vi "Error - Log.vi"(8 "error in (no error)":errorcluster, 11 "Error Data":T1) -> (0 "error out":errorcluster)   [LabVIEW 2017]
doc: "Maintainance a error log file\n[Covers: EH4]"
uses:
  Controls/Error Data.ctl
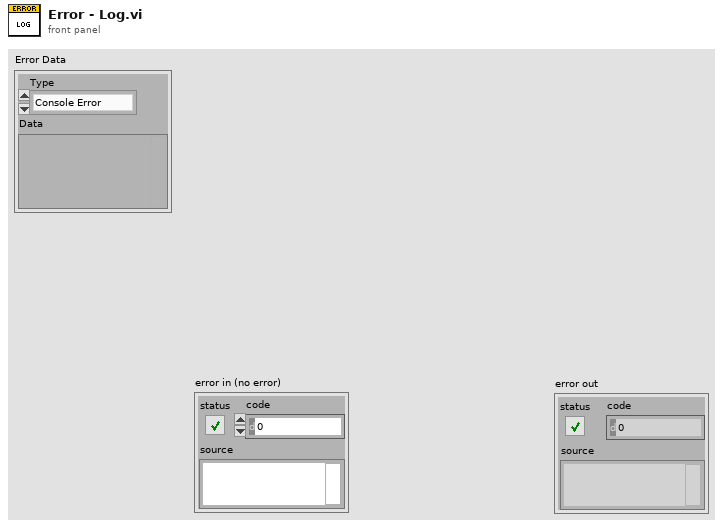
[diagram p1: front panel]
types:
  T1 = typedef "Error Data.ctl" = cluster{"Type":enum16{"Console Error", "Sensor Interface IO Error", "Process Step Error"}, "Data":variant}
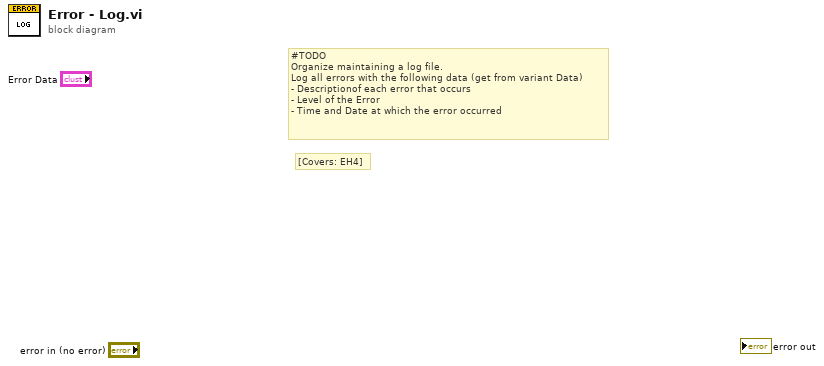
[diagram p0: block diagram]
diagram:
  # "[Covers: EH4]"
  # "#TODO\nOrganize maintaining a log file.\nLog all errors with the following data (get from variant Data)\n- Descriptionof each error that occurs\n- Level of the Error\n- Time and Date at which the error occurred"
